vi "Clear FIFO Error.vi"(8 "error in (no error)":errorcluster) -> (0 "error out":errorcluster)   [LabVIEW 2017]
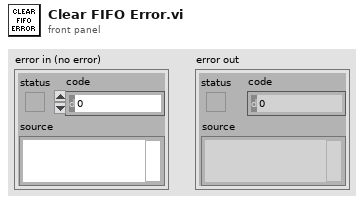
[diagram p1: front panel]
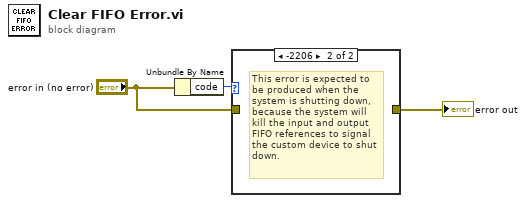
[diagram p0: block diagram]
diagram:
  n1 = Unbundle By Name("error in (no error)") -> ("code"=w3:i32)
  n2 = case shown="-2206" w3 {
    tunnel: [w4 _] -> w1
    tunnel: "error in (no error)" -> [w4 _]
    frame 0, Default {
    }
    frame -2206 {
      # "This error is expected to be produced when the system is shutting down, because the system will kill the input and output FIFO references to signal the custom device to shut down."
    }
  }
  "error out" <- w1
